vi "Close.vi"(8 "error in (no error)":errorcluster) -> (0 "error out":errorcluster)   [LabVIEW 2018, in "text_file.lvlib"]
doc: "Closes the reference to the text file."
uses:
  text_file.lvlib
  private_data (library_variable).vi
panel:
  # "Development\ncontrols/indicators useful for development and testing, but which are not outputs of the VI"
  # "Input\nInputs to the VI"
  # "Output\nOutputs of the VI"
  # "Description\n\nBlank VI with error handling case. \n\nSummarize the use of this VI in this space."
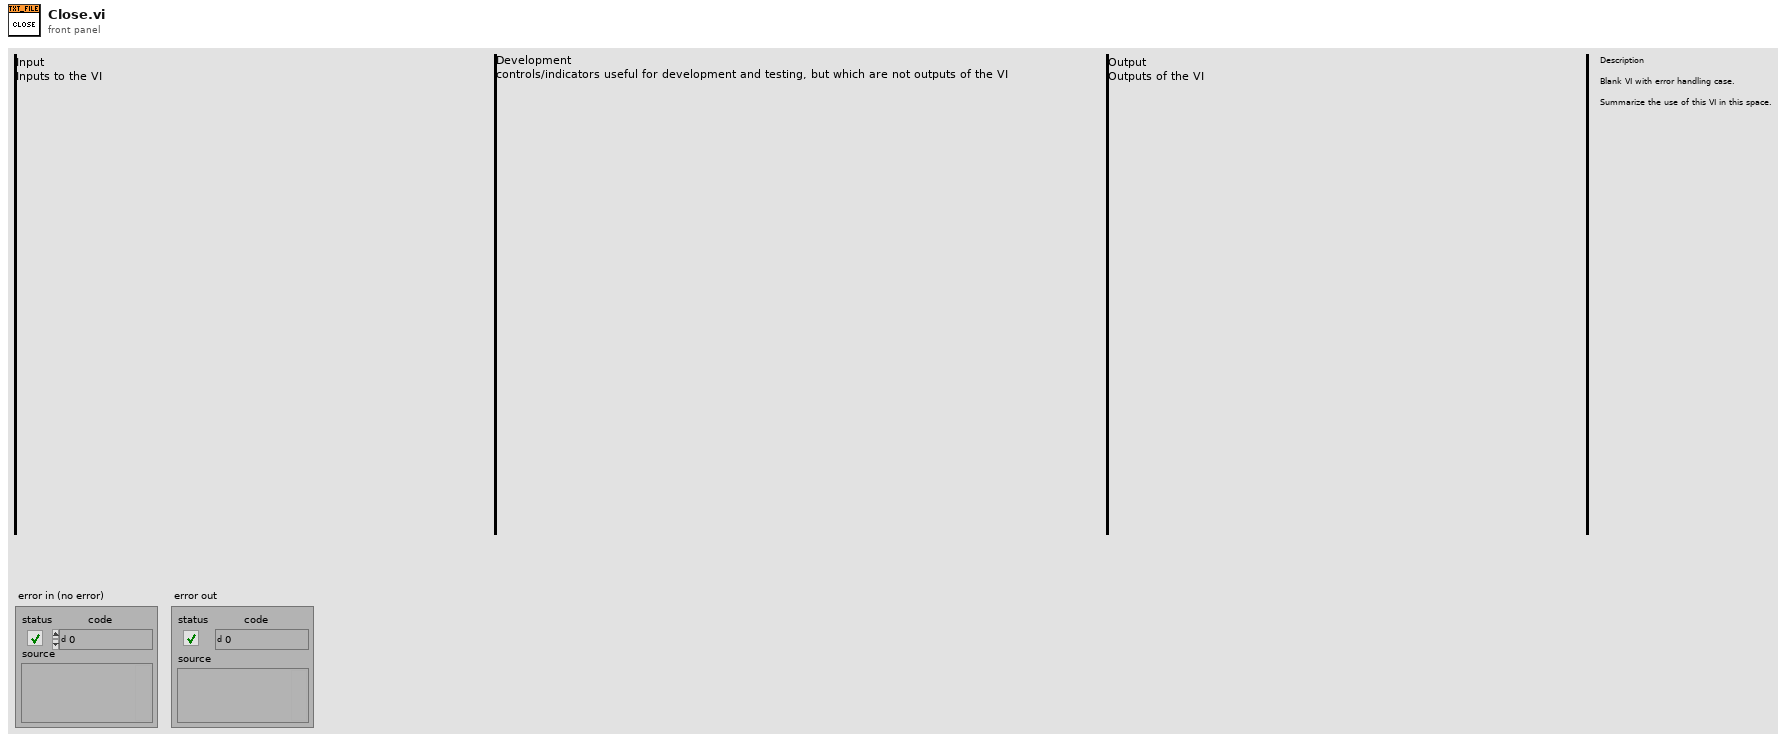
[diagram p1: front panel]
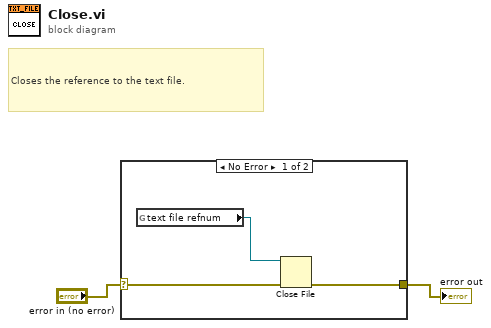
[diagram p0: block diagram]
diagram:
  # "Closes the reference to the text file."
  n1 = case shown="No Error" "error in (no error)" {
    selector: "error in (no error)" -> [w5 w6]
    tunnel: [w4 w6] -> w1
    frame No Error {
      n2 = global read "private_data (library_variable).vi" "text file refnum"() -> (w3:refnum<file>)
      n3 = Close File(refnum=w3, error in=w5) -> (error out=w4:errorcluster)  [unwired: 1 out]
    }
    frame Error {
    }
  }
  "error out" <- w1
